vi "FGV-BroadcastRegistry.vi"(0 "Source":string, 5 "Target":string, 7 "Status":string, 9 "API":string, 11 "Error in":errorcluster caption="Error in (no error)", 12 "Operation":T1) -> (4 "response message":string[](array[string]), 15 "Error out":errorcluster)   [LabVIEW 2020, in "Communicable State Machine.lvlib"]
uses:
  Communicable State Machine.lvlib
  Operation-BroadcastRegistry.ctl
  BroadcastRegistry.lvclass
  global-Broadcast Cache Change Flag.vi
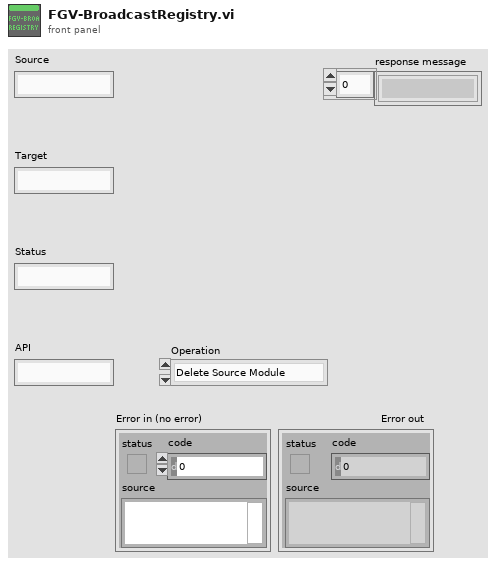
[diagram p1: front panel]
types:
  T1 = typedef "Communicable State Machine.lvlib/Operation-BroadcastRegistry.ctl" = enum16{"Delete Source Module", "Delete Target Module", "Remove Module", "Register", "Unregister", "Check", "List Status", "List Entries"}
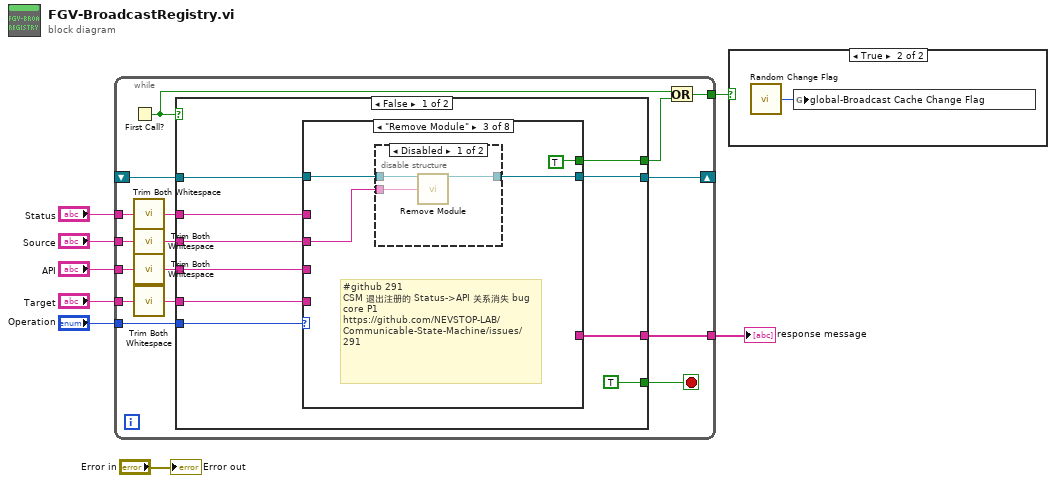
[diagram p0: block diagram]
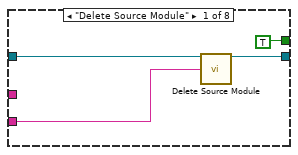
[diagram p2: hidden frame]
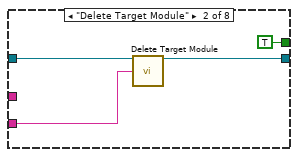
[diagram p3: hidden frame]
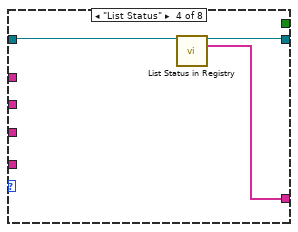
[diagram p5: hidden frame]
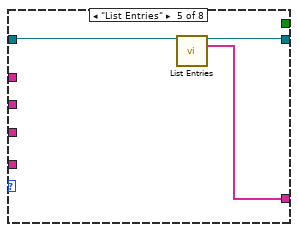
[diagram p6: hidden frame]
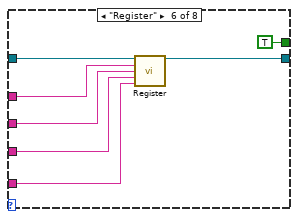
[diagram p7: hidden frame]
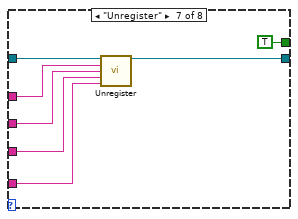
[diagram p8: hidden frame]
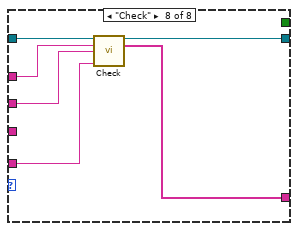
[diagram p9: hidden frame]
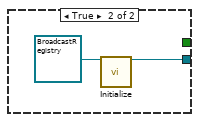
[diagram p10: hidden frame]
diagram:
  n1 = while {
    shift-right: [w23] -> _
    shift-left: _ -> [w22]
    tunnel: "Operation" -> [w21]
    tunnel: "Target" -> [w14]
    tunnel: "Source" -> [w13]
    tunnel: "Status" -> [w15]
    tunnel: "API" -> [w16]
    tunnel: [w20] -> w3
    tunnel: [w17] -> w1
    stop <- w24 stop-if-true
    n2 = First Call?() -> (First Call?: T/F=w18:bool)
    n3 = call "Trim Both Whitespace.vi"("string"=w15) -> ("trimmed string"=w10:string)  [unwired: 1 in]
    n4 = call "Trim Both Whitespace.vi"("string"=w13) -> ("trimmed string"=w12:string)  [unwired: 1 in]
    n5 = call "Trim Both Whitespace.vi"("string"=w16) -> ("trimmed string"=w9:string)  [unwired: 1 in]
    n6 = call "Trim Both Whitespace.vi"("string"=w14) -> ("trimmed string"=w11:string)  [unwired: 1 in]
    n7 = case shown="False" w18 {
      tunnel: [TRUE _] -> w24
      tunnel: [w25 w77] -> w23
      tunnel: w22 -> [w26 _]
      tunnel: w21 -> [w33 _]
      tunnel: w11 -> [w32 _]
      tunnel: w12 -> [w31 _]
      tunnel: w10 -> [w30 _]
      tunnel: w9 -> [w29 _]
      tunnel: [w28 _] -> w20
      tunnel: [w27 _] -> w19
      frame False {
        n8 = case shown="\"Remove Module\"" w33 {
          tunnel: [w36 w40 w44 w52 w55 w62 w68 w75] -> w25
          tunnel: w26 -> [w37 w41 w45 w53 w56 w61 w69 w76]
          tunnel: w32 -> [_ _ _ _ _ w57 w65 w73]
          tunnel: w31 -> [w35 w39 w43 _ _ w59 w66 w72]
          tunnel: w30 -> [_ _ _ _ _ w60 w67 w71]
          tunnel: w29 -> [_ _ _ _ _ w58 w64 _]
          tunnel: [_ _ _ w51 w54 _ _ w74] -> w28
          tunnel: [TRUE ("Cache changed?") TRUE ("Cache changed?") TRUE ("Cache changed?") _ _ TRUE ("Cache changed?") TRUE ("Cache changed?") _] -> w27
          frame "Delete Source Module" {
            n9 = call "Delete Source Module.vi"("BroadcastRegistry in"=w37, "Source"=w35) -> ("BroadcastRegistry out"=w36:refnum<class "BroadcastRegistry.lvclass">)  [unwired: 13 in]
          }
          frame "Delete Target Module" {
            n10 = call "Delete Target Module.vi"("BroadcastRegistry in"=w41, "Source"=w39) -> ("BroadcastRegistry out"=w40:refnum<class "BroadcastRegistry.lvclass">)  [unwired: 13 in]
          }
          frame "Remove Module" {
            # "#github 291\nCSM 退出注册的 Status->API 关系消失 bug core P1\nhttps://github.com/NEVSTOP-LAB/Communicable-State-Machine/issues/291"
            n11 = disable-structure shown="Disabled" {
              disable-tunnel: w45 -> [w49 w50]
              disable-tunnel: [w48 w50] -> w44
              disable-tunnel: w43 -> [w47 _]
              frame Disabled {
                n12 = call "Remove Module.vi"("BroadcastRegistry in"=w49, "Source"=w47) -> ("BroadcastRegistry out"=w48:refnum<class "BroadcastRegistry.lvclass">)  [unwired: 13 in]
              }
              frame Enabled {
              }
            }
          }
          frame "List Status" {
            n13 = call "List Status in Registry.vi"("BroadcastRegistry in"=w53) -> ("BroadcastRegistry out"=w52:refnum<class "BroadcastRegistry.lvclass">, "Status"=w51:string[])  [unwired: 13 in]
          }
          frame "List Entries" {
            n14 = call "List Entries.vi"("BroadcastRegistry in"=w56) -> ("BroadcastRegistry out"=w55:refnum<class "BroadcastRegistry.lvclass">, "Array"=w54:string[])  [unwired: 13 in]
          }
          frame "Register" {
            n15 = call "Register.vi"("BroadcastRegistry in"=w61, "status"=w60, "source"=w59, "api"=w58, "target"=w57) -> ("BroadcastRegistry out"=w62:refnum<class "BroadcastRegistry.lvclass">)  [unwired: 10 in]
          }
          frame "Unregister" {
            n16 = call "Unregister.vi"("BroadcastRegistry in"=w69, "Status"=w67, "Source"=w66, "api"=w64, "Target"=w65) -> ("BroadcastRegistry out"=w68:refnum<class "BroadcastRegistry.lvclass">)  [unwired: 10 in]
          }
          frame "Check" {
            n17 = call "Check.vi"("BroadcastRegistry in"=w76, "Status"=w71, "Source"=w72, "Target"=w73) -> ("BroadcastRegistry out"=w75:refnum<class "BroadcastRegistry.lvclass">, "Response Message Info"=w74:string[])  [unwired: 10 in]
          }
        }
      }
      frame True {
        n18 = call "Initialize.vi"("BroadcastRegistry in"=refnum<class "BroadcastRegistry.lvclass"> refnum ("BroadcastRegistry.lvclass")) -> ("BroadcastRegistry out"=w77:refnum<class "BroadcastRegistry.lvclass">)  [unwired: 14 in]
      }
    }
    n19 = Or(x=w18, y=w19) -> (x .or. y?=w17:bool)
  }
  "response message" <- w3
  n20 = case shown="True" w1 {
    frame False {
    }
    frame True {
      n21 = call "Random Change Flag.vi"() -> ("Random Change Flag"=w79:u64)  [unwired: 2 in]
      n22 = global write "global-Broadcast Cache Change Flag.vi" "global-Broadcast Cache Change Flag"(w79) -> ()
    }
  }
  "Error out" <- "Error in"
